vi "Process.vi"(8 "error in":errorcluster, 11 "SMO.UI.ByRefWithEvents":refnum<class "SMO.UI.Basic.lvclass">) -> (0 "error out":errorcluster, 3 "SMO.UI.ByRefWithEvents out":refnum<class "SMO.UI.Basic.lvclass">)   [LabVIEW 2019, in "SMO.UI.Basic.lvclass"]
doc: "---------------------------------------------------------------\nJKI State Machine Objects™\nhttp://jki.net/state-machine-objects/\nCopyright (C) 2005-2015, JKI <info@jki.net>\nALL RIGHTS RESERVEDJKI State Machine Objects (SMO) 1.0.0.5\nJKI - JKI\nCopyright (c) 2016, JKI"
uses:
  SMO.UI.Basic.lvclass
  C:/Users/Patrick/Documents/GitHub/Test (LV2019)/lv-venv/lv.lib/vi.lib/JKI/JKI SMO/SMO/SMO.lvclass
  C:/Users/Patrick/Documents/GitHub/Test (LV2019)/lv-venv/lv.lib/vi.lib/JKI/JKI SMO/SMO.UI/SMO.UI.lvclass
  vi.lib/JKI/JKI SMO/SMO/Typedefs/Parent Call--Enum.ctl
  vi.lib/JKI/JKI SMO/SMO.UI/SMO.UI.lvclass
  vi.lib/JKI/JKI SMO/SMO/SMO.lvclass
panel:
  # "For instructions on how to use the JKI State Machine Objects, examples and video tutorials, visit:\nhttp://jki.net/state-machine-objects/\n\nJKI State Machine Objects™\nhttp://jki.net/state-machine-objects/\nCopyright (C) 2005-2015, JKI <info@jki.net>\nALL RIGHTS RESERVED"
  # "SMO UI Template"
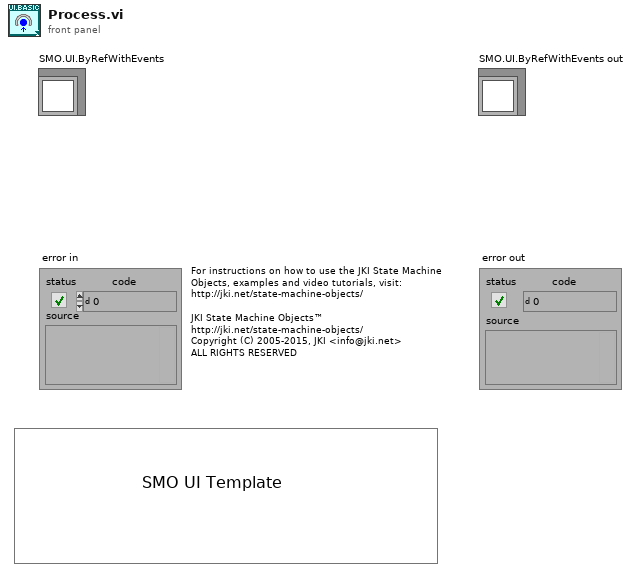
[diagram p1: front panel]
types:
  T1 = typedef "SMO.lvclass/Parent Call--Enum.ctl" = enum16{"Allows parent to run", "Does not request parent to run"}
  T2 = enum32{"invalid app kind", "Development System", "Run Time System", "Student Edition", "Embedded LabVIEW", "Evaluation", "Custom"}
  T3 = enum32{"Invalid", "Standard", "Closed", "Hidden", "Minimized", "Maximized"}
  T4 = cluster{"Core":cluster{"Current VI Reference":refnum<vi>, "Close Panel on Exit?":bool, "error":errorcluster}, "Self Reference":refnum<class "SMO.UI.Basic.lvclass">, "Your string data":string}
  T5 = cluster{"Current VI Reference":refnum<vi>, "Close Panel on Exit?":bool, "error":errorcluster}
  T6 = typedef "SMO.lvclass/Protected Events.ctl" = cluster{"StopProcesses":refnum<user-event>, "AbortProcesses":refnum<user-event>, "Config Changed":refnum<user-event>, "Dependency":refnum<user-event>}
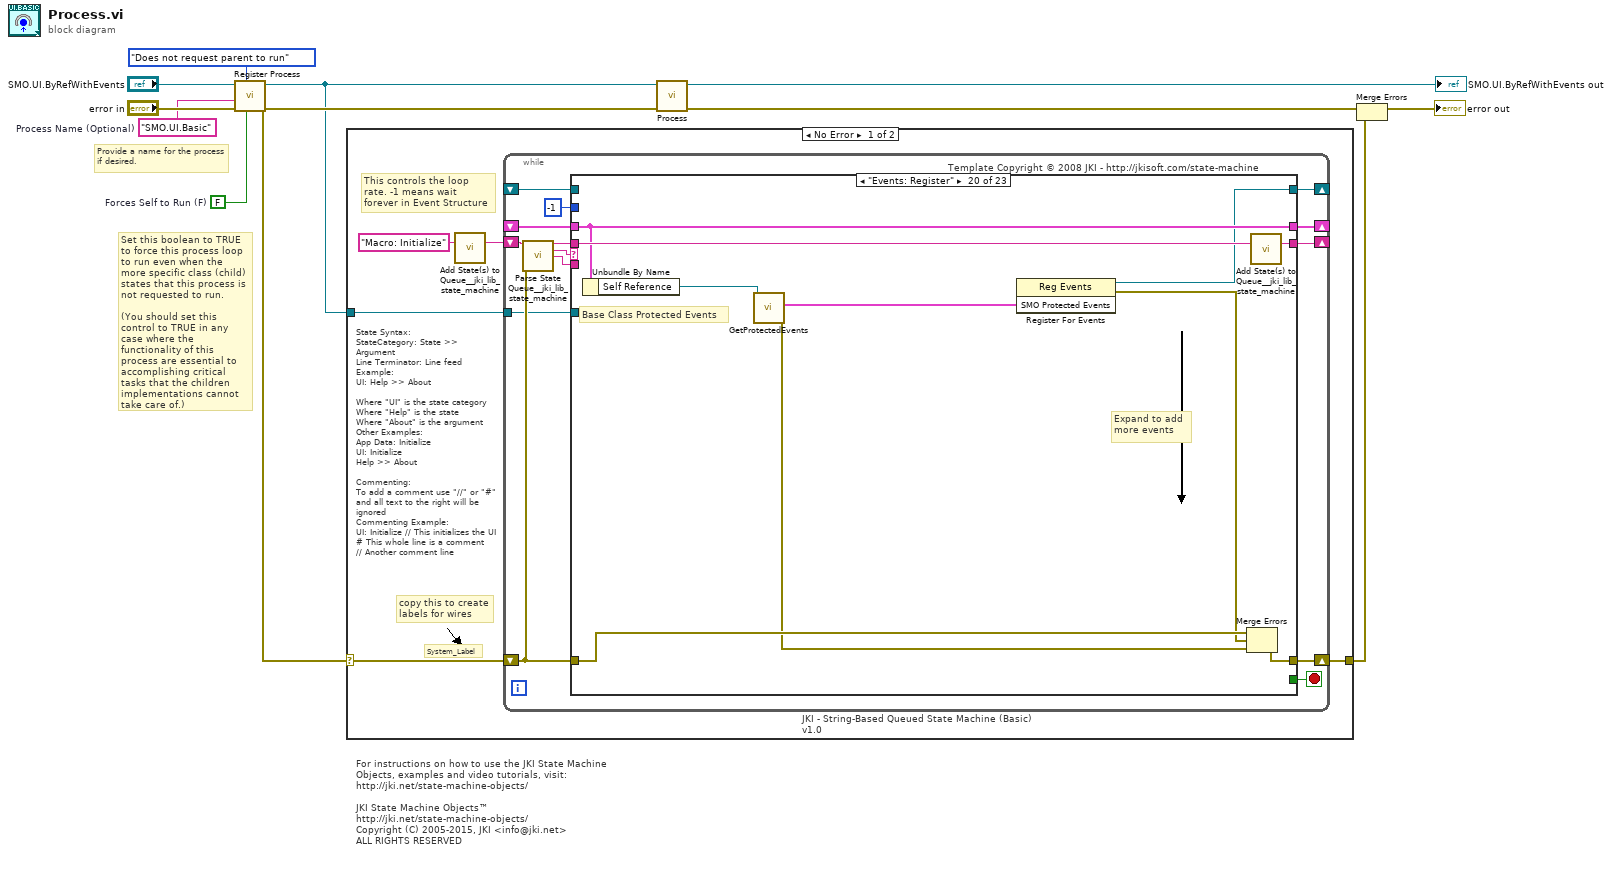
[diagram p0: block diagram]
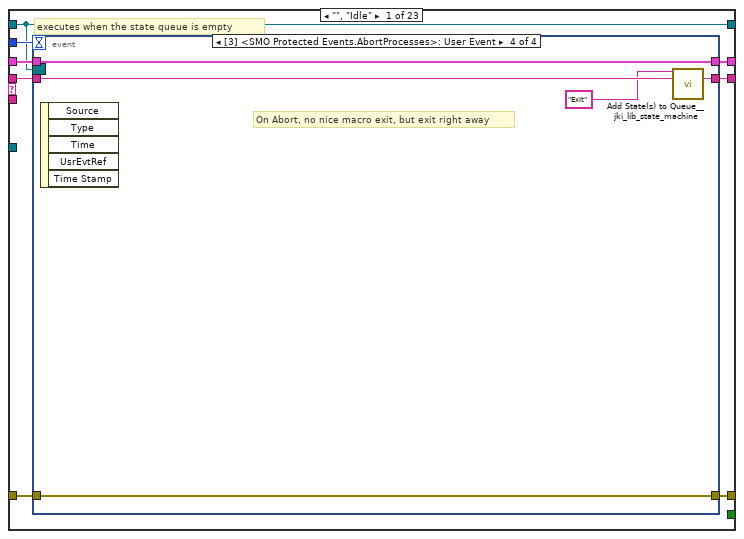
[diagram p2: hidden frame]
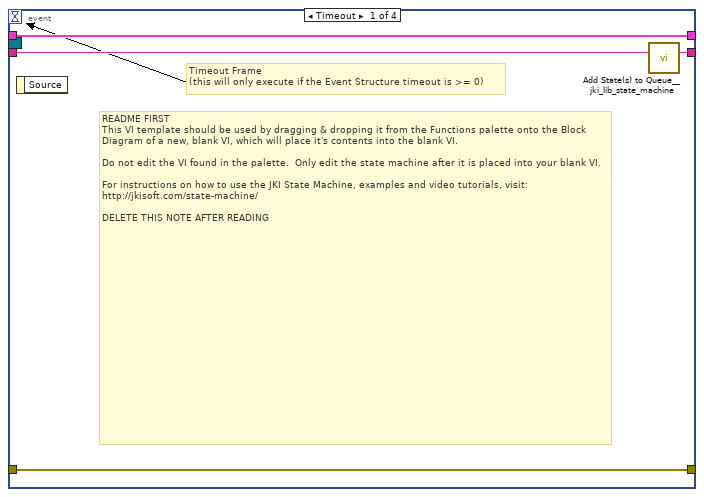
[diagram p3: hidden frame]
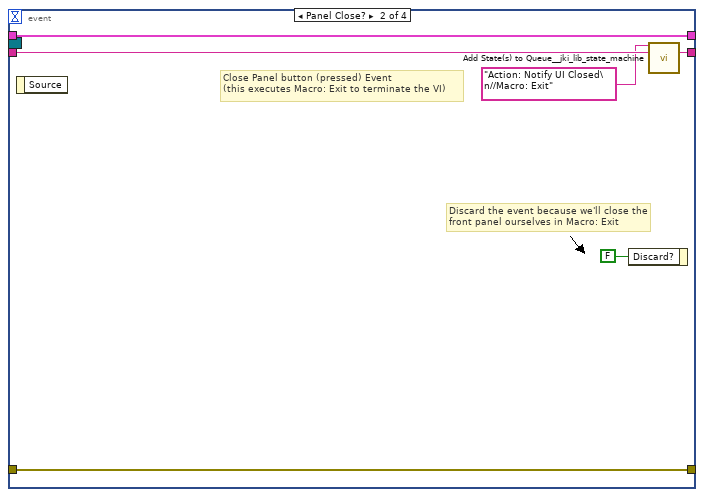
[diagram p4: hidden frame]
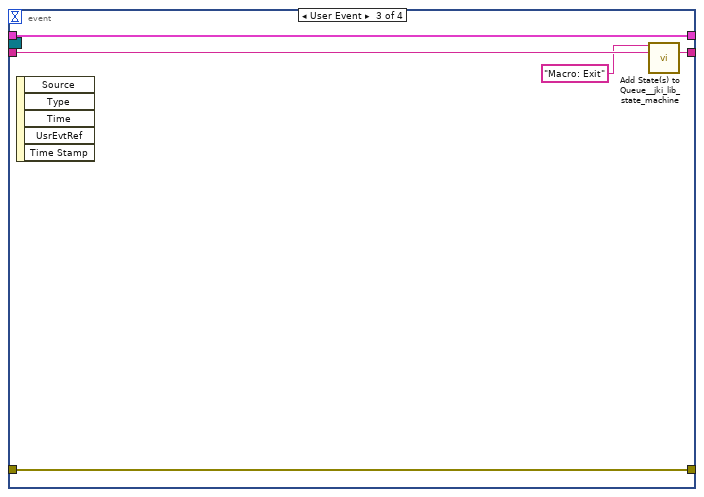
[diagram p5: hidden frame]
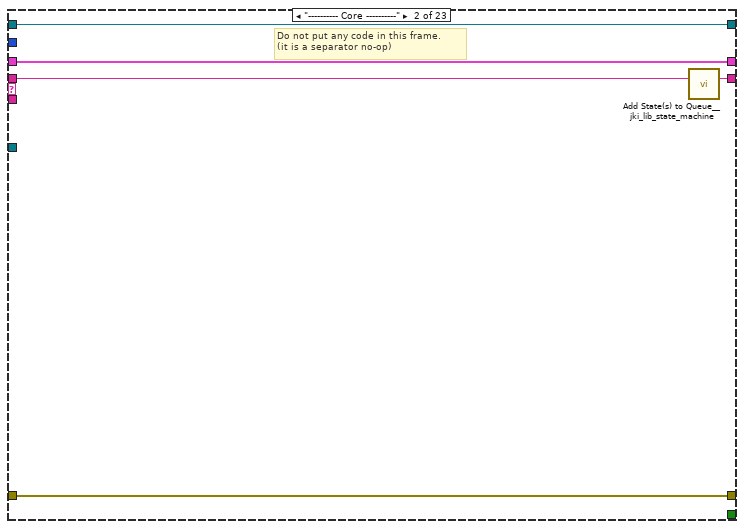
[diagram p6: hidden frame]
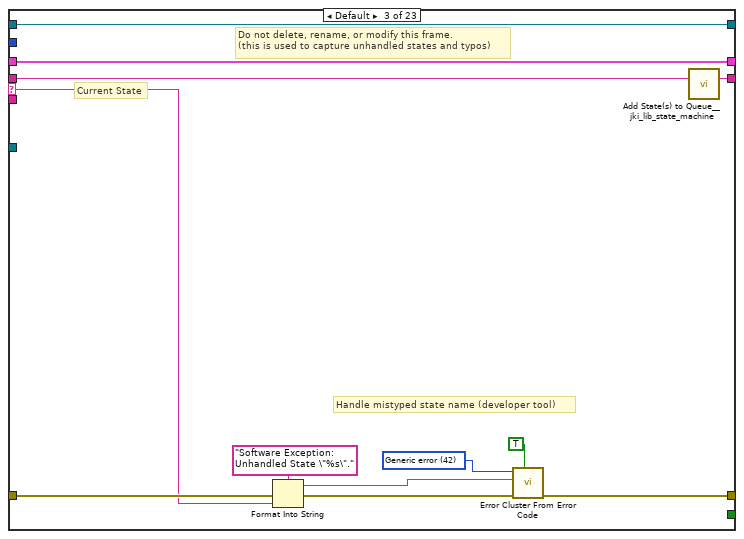
[diagram p7: hidden frame]
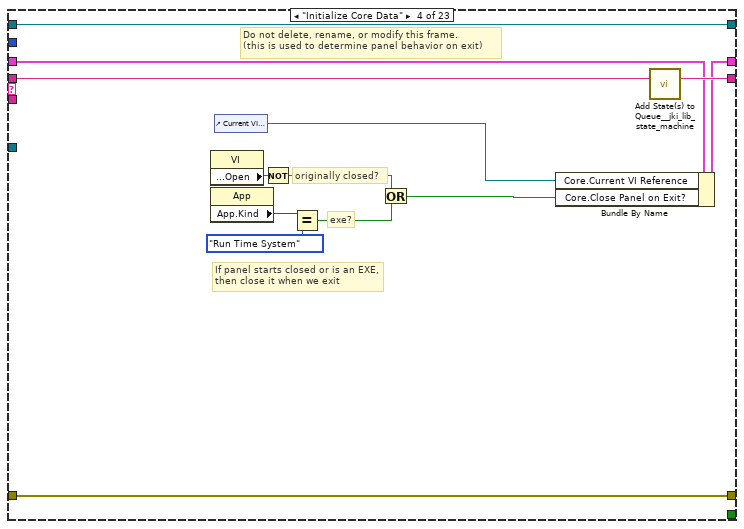
[diagram p8: hidden frame]
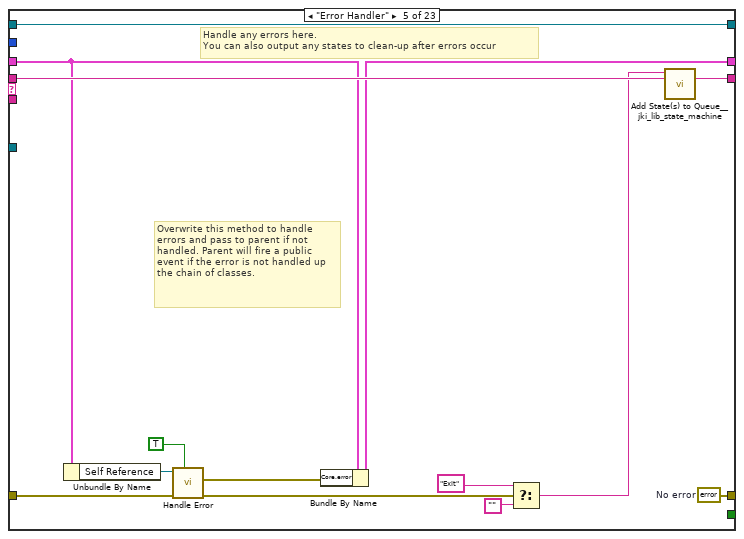
[diagram p9: hidden frame]
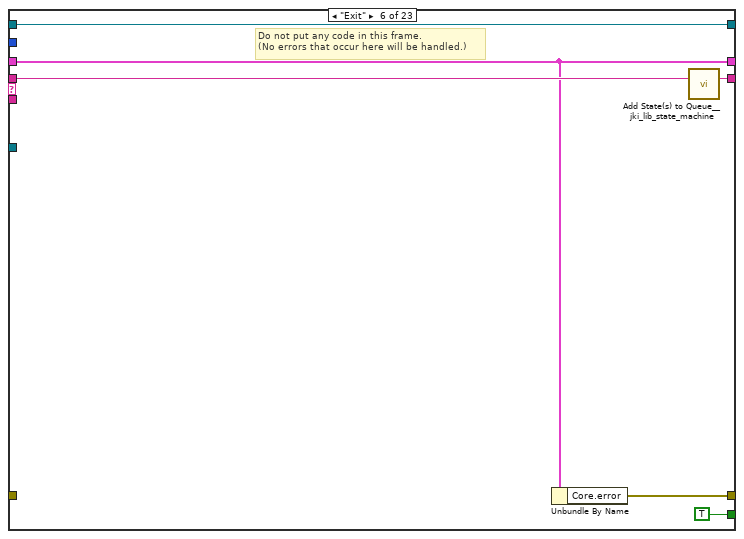
[diagram p10: hidden frame]
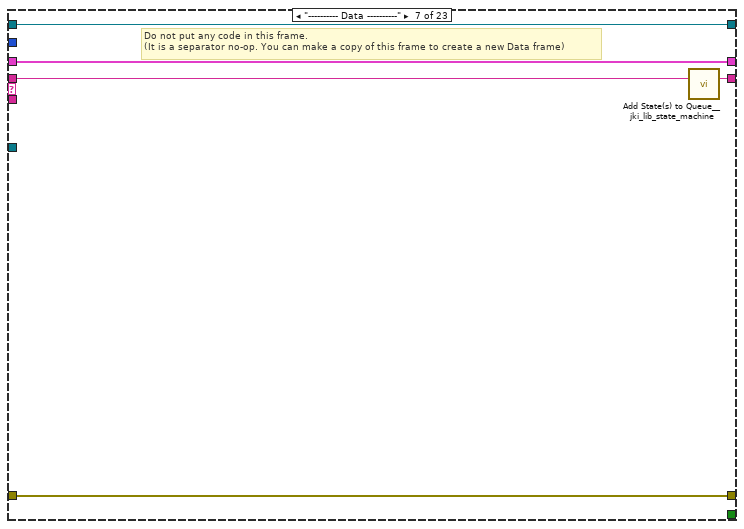
[diagram p11: hidden frame]
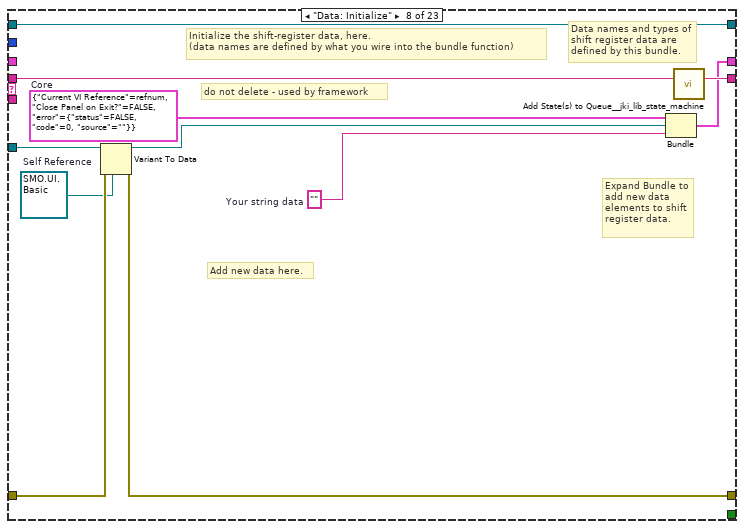
[diagram p12: hidden frame]
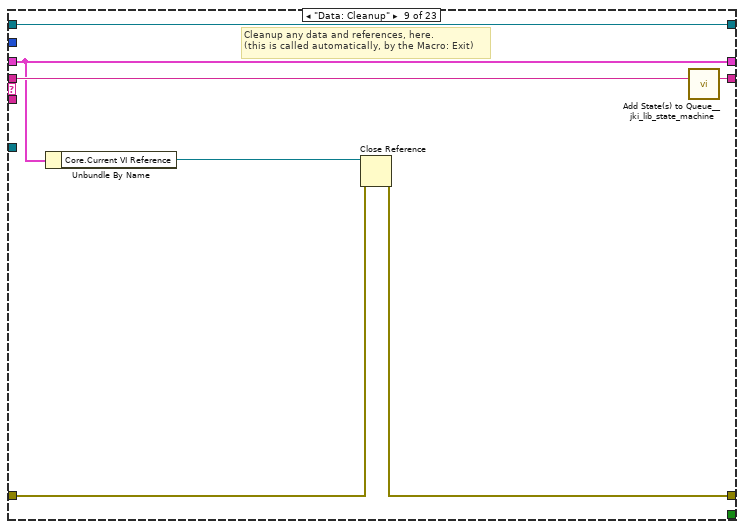
[diagram p13: hidden frame]
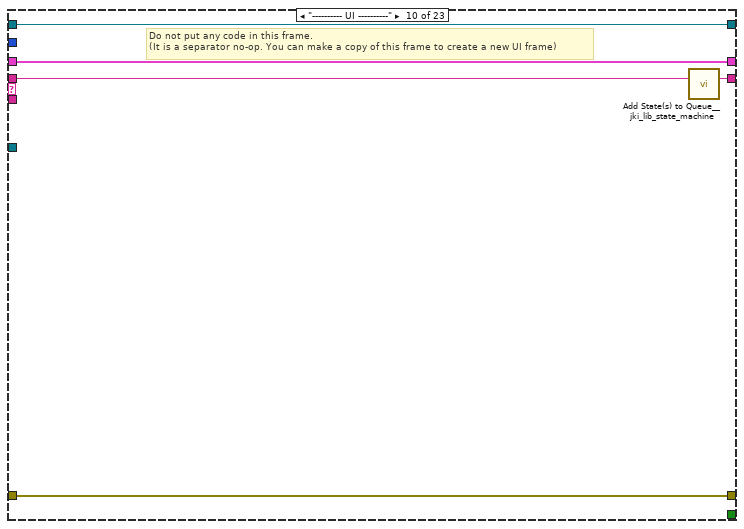
[diagram p14: hidden frame]
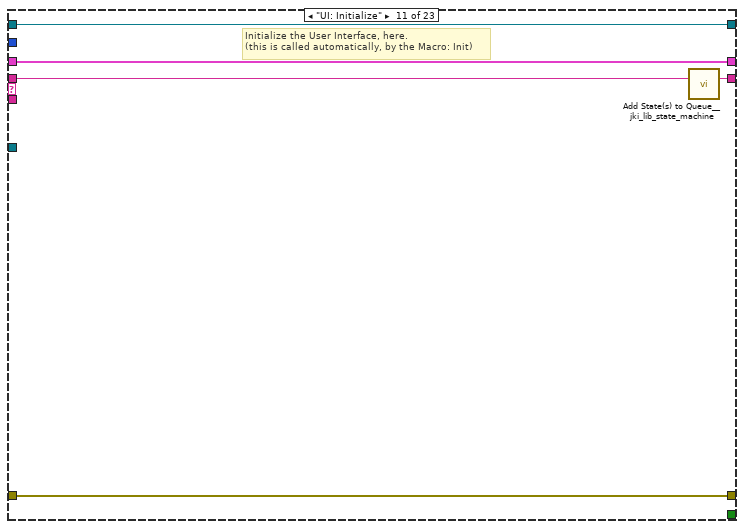
[diagram p15: hidden frame]
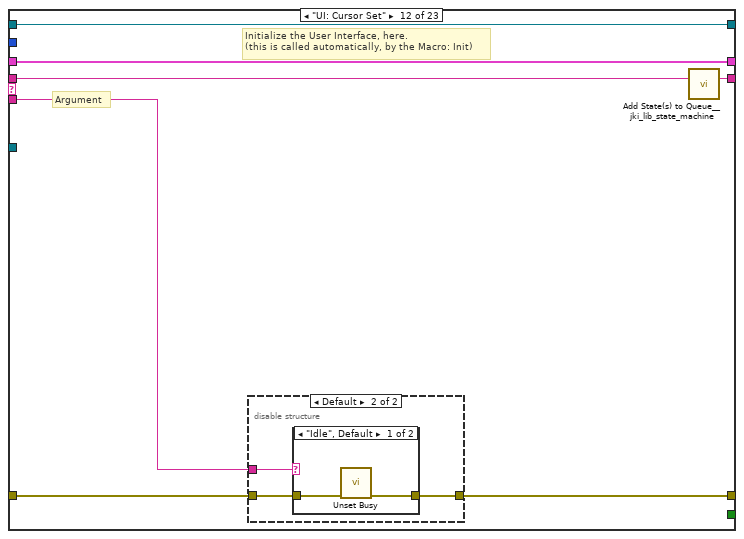
[diagram p16: hidden frame]
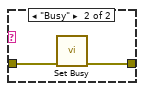
[diagram p18: hidden frame]
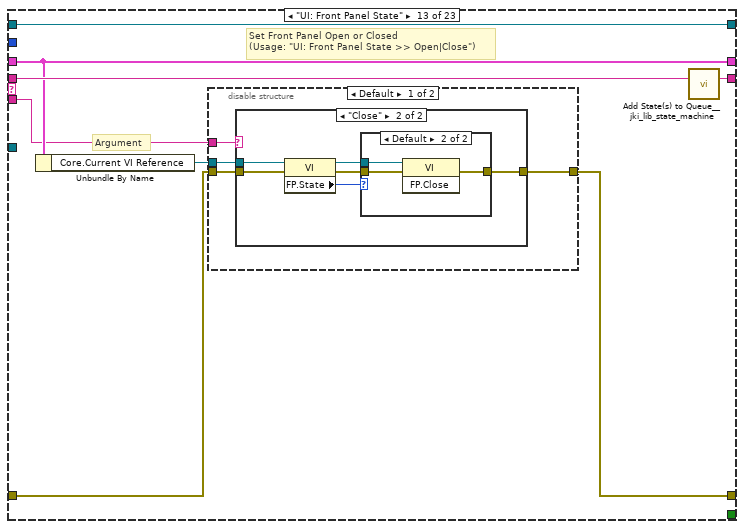
[diagram p19: hidden frame]
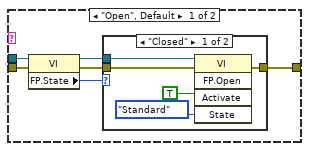
[diagram p20: hidden frame]
diagram:
  w2 = FALSE  # Forces Self to Run (F)
  w1 = "SMO.UI.Basic"  # Process Name (Optional)
  # "Provide a name for the process\nif desired."
  # "Set this boolean to TRUE to force this process loop to run even when the more specific class (child) states that this process is not requested to run.\n\n(You should set this control to TRUE in any case where the functionality of this process are essential to accomplishing critical tasks that the children implementations cannot take care of.)"
  # "For instructions on how to use the JKI State Machine Objects, examples and video tutorials, visit:\nhttp://jki.net/state-machine-objects/\n\nJKI State Machine Objects™\nhttp://jki.net/state-machine-objects/\nCopyright (C) 2005-2015, JKI <info@jki.net>\nALL RIGHTS RESERVED"
  n1 = call "Register Process.vi"("Forces Self to Run (F)"=w2, "Parent Call"=Parent_Call--Enum."Does not request parent to run", "error in (no error)"="error in", "Process Name (optional)"=w1, "SMO"="SMO.UI.ByRefWithEvents") -> ("error out"=w8:errorcluster, "SMO out"=w7:refnum<class "SMO.UI.Basic.lvclass">)  [unwired: 5 in]
  n2 = case shown="No Error" w8 {
    selector: w8 -> [w13 w271]
    tunnel: w7 -> [w14 _]
    tunnel: [w12 w271] -> w4
    frame No Error {
      # "State Syntax:\nStateCategory: State >> Argument\nLine Terminator: Line feed\nExample:\nUI: Help >> About\n\nWhere \"UI\" is the state category\nWhere \"Help\" is the state\nWhere \"About\" is the argument\nOther Examples:\nApp Data: Initialize\nUI: Initialize\nHelp >> About\n\nCommenting:\nTo add a comment use \"//\" or \"#\" and all text to the right will be ignored\nCommenting Example:\nUI: Initialize // This initializes the UI\n# This whole line is a comment\n// Another comment line"
      # "copy this to create labels for wires"
      # "This controls the loop rate. -1 means wait forever in Event Structure"
      # "System_Label"
      n3 = call "Add State(s) to Queue__jki_lib_state_machine.vi"("State(s) in (\"\")"="Macro: Initialize") -> ("States Out"=w16:string)  [unwired: 14 in]
      n4 = while "JKI - String-Based Queued State Machine (Basic) v1.0" {
        shift-right: [w23] -> _
        shift-left: _ -> [w22]
        shift-right: [w26] -> w12
        shift-left: w13 -> [w20]
        shift-right: [w25] -> _
        shift-left: w16 -> [w27]
        tunnel: w14 -> [w19]
        shift-right: [w18] -> _
        shift-left: _ -> [w17]
        stop <- w24 stop-if-true
        # "Template Copyright © 2008 JKI - http://jkisoft.com/state-machine"
        n5 = call "Parse State Queue__jki_lib_state_machine.vi"("State Queue"=w27, "Error In (no error)"=w20) -> ("Remaining States"=w29:string, "Current State"=w30:string, "Arguments"=w28:string)  [unwired: 11 in]
        n6 = case shown="\"Events: Register\"" w30 {
          selector: w30 -> [_ _ w65 _ _ _ _ _ _ _ _ _ _ _ _ _ _ _ _ _ _ _ _]
          tunnel: w29 -> [w38 w63 w69 w88 w102 w108 w113 w124 w131 w136 w141 w148 w164 w196 w205 w219 w224 w235 w240 w250 w256 w263 w270]
          tunnel: w28 -> [_ _ _ _ _ _ _ _ _ _ _ w142 w158 _ _ _ _ _ _ _ _ _ _]
          tunnel: w22 -> [w36 w60 w67 w79 w91 w104 w110 _ w126 w133 w139 w146 w160 w193 w201 w210 w221 w232 w237 w248 w254 w259 w266]
          tunnel: [w35 w61 w71 w85 w93 w103 w111 w119 w127 w134 w138 w143 w161 w194 w203 w217 w222 w226 w238 w242 w251 w260 w264] -> w26
          tunnel: w20 -> [w34 w61 w70 w85 w98 _ w111 w120 w128 w134 w138 w144 w162 w194 w203 w217 w222 w227 w238 w244 w252 w260 w265]
          tunnel: [w37 w62 w68 w87 w101 w107 w112 w123 w130 w135 w140 w147 w163 w195 w204 w218 w223 w234 w239 w249 w255 w262 w269] -> w25
          tunnel: [_ _ _ _ _ TRUE _ _ _ _ _ _ _ _ _ _ _ _ _ _ _ _ _] -> w24
          tunnel: [w33 w60 w67 w86 w90 w104 w110 w122 w126 w133 w139 w146 w160 w193 w201 w210 w221 w232 w237 w248 w254 w258 w266] -> w23
          tunnel: -1 ("Timeout") -> [w32 _ _ _ _ _ _ _ _ _ _ _ _ _ _ _ _ _ _ _ _ _ _]
          tunnel: w19 -> [_ _ _ _ _ _ _ w117 _ _ _ _ _ _ _ _ _ _ _ _ _ _ _]
          tunnel: [w31 w59 w64 w76 w100 w105 w109 w115 w125 w132 w137 w145 w157 w192 w202 w211 w220 w233 w236 w247 w253 w261 w268] -> w18
          tunnel: w17 -> [w31 w59 w64 w76 w100 w105 w109 w115 w125 w132 w137 w145 w157 w192 w202 w211 w220 w233 w236 _ w253 w261 w268]
          frame "", "Idle" {
            # "executes when the state queue is empty"
            n7 = event shown="[3] <SMO Protected Events.AbortProcesses>: User Event" {
              selector: w31 -> [_ _ _ _]
              dyn-events: _ -> [_ _ _ _]
              timeout: w32 -> [_ _ _ _]
              tunnel: w38 -> [w42 w48 w53 w58]
              tunnel: [w41 w47 w52 w57] -> w37
              tunnel: w36 -> [w39 w44 w50 w55]
              tunnel: [w40 w43 w51 w56] -> w35
              tunnel: w34 -> [w40 w43 w51 w56]
              tunnel: [w39 w44 w50 w55] -> w33
              event Timeout {
                # "README FIRST\nThis VI template should be used by dragging & dropping it from the Functions palette onto the Block Diagram of a new, blank VI, which will place it's contents into the blank VI.\n\nDo not edit the VI found in the palette.  Only edit the state machine after it is placed into your blank VI.\n\nFor instructions on how to use the JKI State Machine, examples and video tutorials, visit:\nhttp://jkisoft.com/state-machine/\n\nDELETE THIS NOTE AFTER READING"
                # "Timeout Frame\n(this will only execute if the Event Structure timeout is >= 0)"
                n8 = event-data() -> ()  [unwired: 1 in, 1 out]
                n9 = call "Add State(s) to Queue__jki_lib_state_machine.vi"("State(s) in (\"\")"=w42) -> ("States Out"=w41:string)  [unwired: 14 in]
              }
              event Panel Close? {
                # "Discard the event because we'll close the front panel ourselves in Macro: Exit"
                # "Close Panel button (pressed) Event\n(this executes Macro: Exit to terminate the VI)"
                n10 = event-data() -> ()  [unwired: 1 in, 1 out]
                n11 = event-data("Discard?"=FALSE) -> ()  [unwired: 1 in, 1 out]
                n12 = call "Add State(s) to Queue__jki_lib_state_machine.vi"("State(s) in Front (\"\")"="Action: Notify UI Closed\n//Macro: Exit", "State(s) in (\"\")"=w48) -> ("States Out"=w47:string)  [unwired: 13 in]
              }
              event User Event {
                n13 = event-data() -> ()  [unwired: 1 in, 5 out]
                n14 = call "Add State(s) to Queue__jki_lib_state_machine.vi"("State(s) in Front (\"\")"="Macro: Exit", "State(s) in (\"\")"=w53) -> ("States Out"=w52:string)  [unwired: 13 in]
              }
              event User Event {
                # "On Abort, no nice macro exit, but exit right away"
                n15 = event-data() -> ()  [unwired: 1 in, 5 out]
                n16 = call "Add State(s) to Queue__jki_lib_state_machine.vi"("State(s) in Front (\"\")"="Exit", "State(s) in (\"\")"=w58) -> ("States Out"=w57:string)  [unwired: 13 in]
              }
            }
          }
          frame "---------- Core ----------" {
            # "Do not put any code in this frame.\n(it is a separator no-op)"
            n17 = call "Add State(s) to Queue__jki_lib_state_machine.vi"("State(s) in (\"\")"=w63) -> ("States Out"=w62:string)  [unwired: 14 in]
          }
          frame Default {
            w74 = 42 items=["No error", "Argument error", "Memory is full", "Out of zone", "End of file", "File already open", "Generic file I/O error", "File not found", "File permission error", "Disk is full", "Duplicate path", "Too many files open", "System feature not enabled", "Resource file not found", "Cannot add resource", "Resource not found", "Image not found", "Image memory error", "Pen does not exist", "Config type invalid", "Config token not found", "Config parse error", "Config memory error", "Bad external code format", "Bad external code offset", "External code not present", "Null window", "Destroy window error", "Null menu", "Print aborted", "Bad print record", "Print driver error", "Windows error during printing", "Memory error during printing", "Print dialog error", "Generic print error", "Invalid device refnum", "Device not found", "Device parameter error", "Device unit error", "Cannot open device", "Device call aborted", "Generic error", "Cancelled by user", "Object ID too low", "Object ID too high", "Object not in heap", "Unknown heap", "Unknown object (invalid DefProc)", "Unknown object (DefProc not in table)", "Message out of range", "Invalid (null) method", "Unknown message", "Manager call not supported", "Bad address", "Network operation in progress", "Network operation timed out", "Connection is busy", "Network attribute not supported", "Network error", "Address in use", "System out of memory", "Connection aborted", "Connection refused", "Not connected", "Already connected", "Connection closed", "Initialization error (interapplication manager)", "Bad occurrence", "Wait on unbound occurrence handler", "Occurrence queue overflow", "Datalog type conflict", "Unused", "Unrecognized type (interapplication manager)", "Memory corrupt", "Failed to make temporary DLL", "Old CIN version", "Drag socket not found", "Failed to load drop-object", "Failed to register OLE object", "Failed to release OLE object", "Format specifier type mismatch", "Unknown format specifier", "Too few format specifiers", "Too many format specifiers", "Scan failed", "Newer CIN version", "Error converting to variant", "Runtime menu error", "Password tampered", "Variant attribute not found", "Incompatible variant data type", "Event data is not available", "Event Store is not present", "Occurrence is not found", "Event Queue is not created", "Event info is not available", "Refnum passed is NULL", "Error retrieving Class GUID", "Error retrieving CoClass GUID", "Error retrieving TypeLib GUID.", "Bad built application magic bytes.", "Specific driver is different from the specific driver associated with the Logical Name.", "There is no session opened to the class driver.", "Max Error", "MAX - Error with config objects", "MAX - Error loading configuration", "MAX - Group not supported"]
            # "Current State"
            # "Do not delete, rename, or modify this frame.\n(this is used to capture unhandled states and typos)"
            # "Handle mistyped state name (developer tool)"
            n18 = Format Into String(format string="Software Exception: Unhandled State \"%s\"." ("message"), error in=w70, w65) -> (resulting string=w73:string, error out=w72:errorcluster)  [unwired: 1 in]
            n19 = call <vilib>:"Error Cluster From Error Code.vi"("show call chain? (False)"=TRUE, "error in (no error)"=w72, "error message (\"\")"=w73, "error code (0)"=w74) -> ("error out"=w71:errorcluster)  [unwired: 5 in]
            n20 = call "Add State(s) to Queue__jki_lib_state_machine.vi"("State(s) in (\"\")"=w69) -> ("States Out"=w68:string)  [unwired: 14 in]
          }
          frame "Initialize Core Data" {
            # "Do not delete, rename, or modify this frame.\n(this is used to determine panel behavior on exit)"
            # "originally closed?"
            # "exe?"
            # "If panel starts closed or is an EXE, then close it when we exit"
            n21 = property class="VI"() -> ("Front Panel.Open"=w84:bool)  [unwired: 2 in, 2 out]
            n22 = property class="App"() -> ("App.Kind"=w83:T2)  [unwired: 2 in, 2 out]
            n23 = control-ref of="Current VI Reference"() -> (w77:refnum<vi>)
            n24 = Not(x=w84) -> (.not. x?=w81:bool)
            n25 = Equal?(x=w83, y=T2."Run Time System" ("Application:Kind")) -> (x = y?=w80:bool)
            n26 = Or(x=w81, y=w80) -> (x .or. y?=w78:bool)
            n27 = Bundle By Name(cluster=w79, "Core.Current VI Reference"=w77, "Core.Close Panel on Exit?"=w78) -> (w86:T4)
            n28 = call "Add State(s) to Queue__jki_lib_state_machine.vi"("State(s) in (\"\")"=w88) -> ("States Out"=w87:string)  [unwired: 14 in]
          }
          frame "Error Handler" {
            w93 = errorcluster {"status"=FALSE, "code"=0, "source"=""}  # No error
            # "Overwrite this method to handle errors and pass to parent if not handled. Parent will fire a public event if the error is not handled up the chain of classes."
            # "Handle any errors here.\nYou can also output any states to clean-up after errors occur"
            n29 = Unbundle By Name(w91) -> ("Self Reference"=w99:refnum<class "SMO.UI.Basic.lvclass">)
            n30 = call-dynamic "Handle Error.vi"("Stop on Unhandled Error (T)"=TRUE, "error in"=w98, "SMO"=w99) -> ("handling error"=w94:errorcluster, "Unhandled error"=w92:errorcluster)  [unwired: 6 in, 1 out]
            n31 = Bundle By Name(cluster=w91, "Core.error"=w92) -> (w90:T4)
            n32 = Select(t="Exit", s=w94, f="") -> (s? t:f=w95:string)
            n33 = call "Add State(s) to Queue__jki_lib_state_machine.vi"("State(s) in Front (\"\")"=w95, "State(s) in (\"\")"=w102) -> ("States Out"=w101:string)  [unwired: 13 in]
          }
          frame "Exit" {
            # "Do not put any code in this frame.\n(No errors that occur here will be handled.)"
            n34 = Unbundle By Name(w104) -> ("Core.error"=w103:errorcluster)
            n35 = call "Add State(s) to Queue__jki_lib_state_machine.vi"("State(s) in (\"\")"=w108) -> ("States Out"=w107:string)  [unwired: 14 in]
          }
          frame "---------- Data ----------" {
            # "Do not put any code in this frame.\n(It is a separator no-op. You can make a copy of this frame to create a new Data frame)"
            n36 = call "Add State(s) to Queue__jki_lib_state_machine.vi"("State(s) in (\"\")"=w113) -> ("States Out"=w112:string)  [unwired: 14 in]
          }
          frame "Data: Initialize" {
            w114 = T5 {"Current VI Reference"=refnum, "Close Panel on Exit?"=FALSE, "error"={"status"=FALSE, "code"=0, "source"=""}}  # Core
            w118 = refnum<class "SMO.UI.Basic.lvclass"> refnum  # Self Reference
            w121 = ""  # Your string data
            # "do not delete - used by framework"
            # "Expand Bundle to add new data elements to shift register data."
            # "Add new data here."
            # "Data names and types of shift register data are defined by this bundle."
            # "Initialize the shift-register data, here.\n(data names are defined by what you wire into the bundle function)"
            n37 = Variant To Data(error in=w120, type=w118, Variant=w117) -> (data=w116:refnum<class "SMO.UI.Basic.lvclass">, error out=w119:errorcluster)
            n38 = Bundle("Core"=w114, "Self Reference"=w116, "Your string data"=w121) -> (w122:T4)  [unwired: 1 in]
            n39 = call "Add State(s) to Queue__jki_lib_state_machine.vi"("State(s) in (\"\")"=w124) -> ("States Out"=w123:string)  [unwired: 14 in]
          }
          frame "Data: Cleanup" {
            # "Cleanup any data and references, here.\n(this is called automatically, by the Macro: Exit)"
            n40 = Unbundle By Name(w126) -> ("Core.Current VI Reference"=w129:refnum<vi>)
            n41 = Close Reference(reference=w129, error in (no error)=w128) -> (error out=w127:errorcluster)
            n42 = call "Add State(s) to Queue__jki_lib_state_machine.vi"("State(s) in (\"\")"=w131) -> ("States Out"=w130:string)  [unwired: 14 in]
          }
          frame "---------- UI ----------" {
            # "Do not put any code in this frame.\n(It is a separator no-op. You can make a copy of this frame to create a new UI frame)"
            n43 = call "Add State(s) to Queue__jki_lib_state_machine.vi"("State(s) in (\"\")"=w136) -> ("States Out"=w135:string)  [unwired: 14 in]
          }
          frame "UI: Initialize" {
            # "Initialize the User Interface, here.\n(this is called automatically, by the Macro: Init)"
            n44 = call "Add State(s) to Queue__jki_lib_state_machine.vi"("State(s) in (\"\")"=w141) -> ("States Out"=w140:string)  [unwired: 14 in]
          }
          frame "UI: Cursor Set" {
            # "Argument"
            # "Initialize the User Interface, here.\n(this is called automatically, by the Macro: Init)"
            n45 = disable-structure shown="Default" {
              disable-tunnel: w144 -> [w149 w152]
              disable-tunnel: [w149 w151] -> w143
              disable-tunnel: w142 -> [_ w150]
              frame condition #0 {
              }
              frame condition #1 (active) {
                n46 = case shown="\"Idle\", Default" w150 {
                  tunnel: w152 -> [w154 w156]
                  tunnel: [w153 w155] -> w151
                  frame "Idle", Default {
                    n47 = call <vilib>:"Unset Busy.vi"("error in (no error)"=w154) -> ("error out"=w153:errorcluster)  [unwired: 10 in]
                  }
                  frame "Busy" {
                    n48 = call <vilib>:"Set Busy.vi"("error in (no error)"=w156) -> ("error out"=w155:errorcluster)  [unwired: 9 in, 1 out]
                  }
                }
              }
            }
            n49 = call "Add State(s) to Queue__jki_lib_state_machine.vi"("State(s) in (\"\")"=w148) -> ("States Out"=w147:string)  [unwired: 14 in]
          }
          frame "UI: Front Panel State" {
            # "Argument"
            # "Set Front Panel Open or Closed\n(Usage: \"UI: Front Panel State >> Open|Close\")"
            n50 = Unbundle By Name(w160) -> ("Core.Current VI Reference"=w159:refnum<vi>)
            n51 = disable-structure shown="Default" {
              disable-tunnel: w162 -> [w168 w191]
              disable-tunnel: [w167 w191] -> w161
              disable-tunnel: w159 -> [w166 _]
              disable-tunnel: w158 -> [w165 _]
              frame condition #0 (active) {
                n52 = case shown="\"Close\"" w165 {
                  tunnel: w168 -> [w172 w185]
                  tunnel: [w174 w186] -> w167
                  tunnel: w166 -> [w173 w183]
                  frame "Open", Default {
                    n53 = property class="VI"(reference=w173, error in=w172) -> (reference out=w170:refnum<vi>, error out=w171:errorcluster, "FP.State"=w169:T3)
                    n54 = case shown="\"Closed\"" w169 {
                      tunnel: [w177 w180] -> w174
                      tunnel: w171 -> [w176 w180]
                      tunnel: w170 -> [w175 _]
                      frame "Closed" {
                        n55 = invoke class="VI" method="FP.Open"(reference=w175, error in=w176, "Activate"=TRUE, "State"=T3."Standard") -> (error out=w177:errorcluster)  [unwired: 1 in, 4 out]
                      }
                      frame Default {
                      }
                    }
                  }
                  frame "Close" {
                    n56 = property class="VI"(reference=w183, error in=w185) -> (reference out=w182:refnum<vi>, error out=w184:errorcluster, "FP.State"=w181:T3)
                    n57 = case shown="Default" w181 {
                      tunnel: [w187 w190] -> w186
                      tunnel: w184 -> [w187 w189]
                      tunnel: w182 -> [_ w188]
                      frame "Invalid", "Closed" {
                      }
                      frame Default {
                        n58 = invoke class="VI" method="FP.Close"(reference=w188, error in=w189) -> (error out=w190:errorcluster)  [unwired: 1 in, 2 out]
                      }
                    }
                  }
                }
              }
              frame condition #1 {
              }
            }
            n59 = call "Add State(s) to Queue__jki_lib_state_machine.vi"("State(s) in (\"\")"=w164) -> ("States Out"=w163:string)  [unwired: 14 in]
          }
          frame "---------- Macro ----------" {
            # "Do not put any code in this frame.\n(It is a separator no-op. You can make a copy of this frame to create a new Macro frame)"
            n60 = call "Add State(s) to Queue__jki_lib_state_machine.vi"("State(s) in (\"\")"=w196) -> ("States Out"=w195:string)  [unwired: 14 in]
          }
          frame "Macro: Initialize" {
            w199 = "UI: Initialize\n//UI: Front Panel State >> Open"  # UI: Initialize //UI: Front Panel State >> Open
            # "Initialization Macro\n(This is called once, when the VI starts)"
            n61 = call "Add State(s) to Queue__jki_lib_state_machine.vi"("State(s) in Front (\"\")"="Data: Initialize\nInitialize Core Data\nEvents: Register", "State(s) in (\"\")"="Process: Sync", "State(s) at Back (\"\")"=w199) -> ("States Out"=w198:string)  [unwired: 12 in]
            n62 = call "Add State(s) to Queue__jki_lib_state_machine.vi"("State(s) in Front (\"\")"=w198, "State(s) in (\"\")"=w205) -> ("States Out"=w204:string)  [unwired: 13 in]
          }
          frame "Macro: Exit" {
            # "Exit Macro\n(This is called once, when the VI exits)"
            n63 = Unbundle By Name(w210) -> ("Core.Close Panel on Exit?"=w216:bool)
            n64 = Select(t="//UI: Front Panel State >> Close", s=w216, f="") -> (s? t:f=w213:string)
            n65 = call "Add State(s) to Queue__jki_lib_state_machine.vi"("State(s) in Front (\"\")"="Data: Cleanup\nEvents: Unregister", "State(s) in (\"\")"="Process: Sync", "State(s) at Back (\"\")"="Exit") -> ("States Out"=w207:string)  [unwired: 12 in]
            n66 = call "Add State(s) to Queue__jki_lib_state_machine.vi"("State(s) in (\"\")"=w213, "State(s) at Back (\"\")"=w207) -> ("States Out"=w212:string)  [unwired: 13 in]
            n67 = call "Add State(s) to Queue__jki_lib_state_machine.vi"("State(s) in Front (\"\")"=w212, "State(s) in (\"\")"=w219) -> ("States Out"=w218:string)  [unwired: 13 in]
          }
          frame "---------- Process ----------" {
            # "Template Separator\n(You can make a copy of, or modify, this frame)"
            n68 = call "Add State(s) to Queue__jki_lib_state_machine.vi"("State(s) in (\"\")"=w224) -> ("States Out"=w223:string)  [unwired: 14 in]
          }
          frame "Process: Sync" {
            n69 = Unbundle By Name(w232) -> ("Self Reference"=w228:refnum<class "SMO.UI.Basic.lvclass">)
            n70 = call "WaitOnProcessSync.vi"("error in (no error)"=w227, "SMO"=w228) -> ("error out"=w226:errorcluster, "Don't run?"=w231:bool)  [unwired: 7 in, 1 out]
            n71 = Select(t="Data: Cleanup\nEvents: Unregister\nExit", s=w231, f="") -> (s? t:f=w225:string)
            n72 = call "Add State(s) to Queue__jki_lib_state_machine.vi"("State(s) in Front (\"\")"=w225, "State(s) in (\"\")"=w235) -> ("States Out"=w234:string)  [unwired: 13 in]
          }
          frame "---------- Events ----------" {
            # "Template Separator\n(You can make a copy of, or modify, this frame)"
            n73 = call "Add State(s) to Queue__jki_lib_state_machine.vi"("State(s) in (\"\")"=w240) -> ("States Out"=w239:string)  [unwired: 14 in]
          }
          frame "Events: Register" {
            # "Expand to add\nmore events"
            # "Base Class Protected Events"
            n74 = Unbundle By Name(w248) -> ("Self Reference"=w245:refnum<class "SMO.UI.Basic.lvclass">)
            n75 = call "GetProtectedEvents.vi"("SMO"=w245) -> ("error out"=w241:errorcluster, "SMO Protected Events"=w246:T6)  [unwired: 8 in, 1 out]
            n76 = register-events(w246) -> (reference out=w247:refnum<event-registration>, error out=w243:errorcluster)  [unwired: 2 in]
            n77 = Merge Errors(w244, w243, w241) -> (w242:errorcluster)
            n78 = call "Add State(s) to Queue__jki_lib_state_machine.vi"("State(s) in (\"\")"=w250) -> ("States Out"=w249:string)  [unwired: 14 in]
          }
          frame "Events: Unregister" {
            n79 = Unregister For Events(event registration refnum=w253, error in=w252) -> (error out=w251:errorcluster)
            n80 = call "Add State(s) to Queue__jki_lib_state_machine.vi"("State(s) in (\"\")"=w256) -> ("States Out"=w255:string)  [unwired: 14 in]
          }
          frame "---------- Action ----------" {
            n81 = Unbundle By Name(w259) -> ("Self Reference"=w257:refnum<class "SMO.UI.Basic.lvclass">)
            n82 = Bundle By Name(cluster=w259, "Self Reference"=w257) -> (w258:T4)
            n83 = call "Add State(s) to Queue__jki_lib_state_machine.vi"("State(s) in (\"\")"=w263) -> ("States Out"=w262:string)  [unwired: 14 in]
          }
          frame "Action: Notify UI Closed" {
            # "Notify that the UI has been closed"
            n84 = Unbundle By Name(w266) -> ("Self Reference"=w267:refnum<class "SMO.UI.Basic.lvclass">)
            n85 = call "Hide.vi"("error in (no error)"=w265, "SMO.UI"=w267) -> ("error out"=w264:errorcluster)  [unwired: 8 in, 1 out]
            n86 = call "Add State(s) to Queue__jki_lib_state_machine.vi"("State(s) in (\"\")"=w270) -> ("States Out"=w269:string)  [unwired: 14 in]
          }
        }
      }
    }
    frame Error {
    }
  }
  n87 = call-parent "Process.vi"("error in (no error)"=w8, "SMO.UI"=w7) -> ("error out"=w5:errorcluster, "SMO.UI out"=→"SMO.UI.ByRefWithEvents out":refnum<class "SMO.UI.Basic.lvclass">)  [unwired: 8 in]
  n88 = Merge Errors(w5, w4) -> (→"error out":errorcluster)
